vi "serialPorts.vi"(8 "list?":bool=TRUE, 11 "Python version":string) -> (0 "error out":errorcluster, 1 "ports":string[](array[string]), 2 "appended path":path, 3 "Refnum out":refnum<k35>)   [LabVIEW 2021]
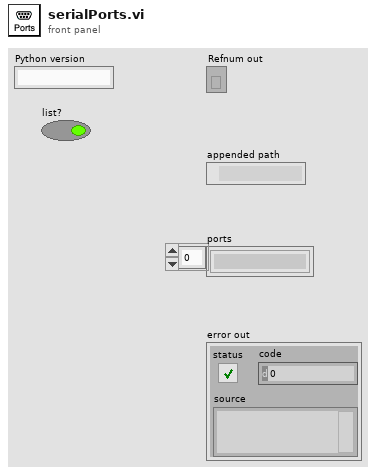
[diagram p1: front panel]
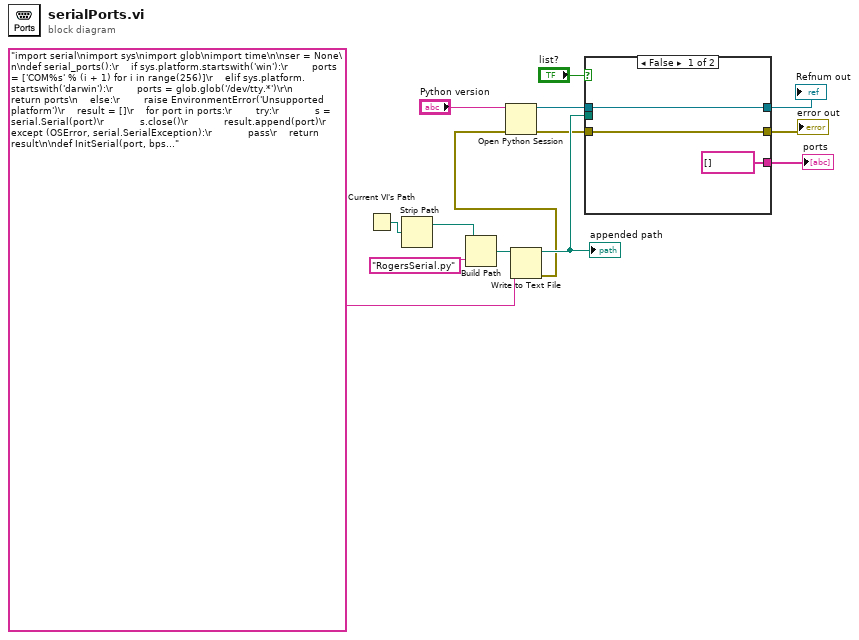
[diagram p0: block diagram]
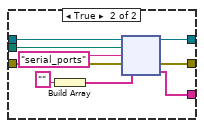
[diagram p2: hidden frame]
diagram:
  n1 = Current VI's Path() -> (path=w7:path)
  n2 = Strip Path(path=w7) -> (stripped path=w8:path)  [unwired: 1 out]
  n3 = Build Path(base path=w8, name or relative path="RogersSerial.py") -> (appended path=w13:path)
  "appended path" <- w13
  n4 = Write to Text File(file (use dialog)=w13, text="import serial\nimport sys\nimport glob\nimport time\n\nser = None\n\ndef serial_ports():\r    if sys.platform.startswith('win'):\r        ports = ['COM%s' % (i + 1) for i in range(256)]\r    elif sys.platform.startswith('darwin'):\r        ports = glob.glob('/dev/tty.*')\r\n        return ports\n    else:\r        raise EnvironmentError('Unsupported platform')\r    result = []\r    for port in ports:\r        try:\r            s = serial.Serial(port)\r            s.close()\r            result.append(port)\r        except (OSError, serial.SerialException):\r            pass\r    return result\n\ndef InitSerial(port, bps = 9600, to = 0):\n    global ser\n    ser = serial.Serial(port, bps, timeout = to)  # open serial port\n    ser.flushInput()\n    ser.flushOutput()\n    return ser.name\n\ndef FlushSerial():\n    ser.flushInput()\n    ser.flushOutput()\n    return(ser.in_waiting)\n\ndef CloseSerial():\n    ser.flush()\n    ser.close()\n    return('done')\n\ndef WriteSerial(string):\n    return (ser.write(string.encode()))    # write a string\n\ndef WriteBytes(data,replyLength):\n    buffer=ser.read(ser.in_waiting)\n    reply = ser.write(bytes(data))\n    if (replyLength < 0): return []\n    return list(ser.read(replyLength))    # write bytes and get reply\n\ndef ScriptSerial(string):\n    reply = ''\n    lines = string.split('\\n')\n    for line in lines:\n        ser.write(line.encode())\n        time.sleep(1)\n        reply += ReadSerial() + '\\n'\n    return reply \n\ndef ReadSerial():\n    reply = ''\n    if ser.in_waiting:\n        reply = ser.readline().decode()\n    return(reply)\n\n# note if the timeout is anything but zero it is slow") -> (error out=w3:errorcluster)  [unwired: 2 in, 2 out]
  n5 = Open Python Session(python version="Python version", 3:w3) -> (session out=w12:refnum<k35>, error out=w2:errorcluster)  [unwired: 1 in]
  n6 = case shown="False" "list?" {
    tunnel: w13 -> [_ w25]
    tunnel: w12 -> [w16 w24]
    tunnel: [w15 w23] -> w11
    tunnel: [string[] [] w22] -> w10
    tunnel: [w16 w18] -> w4
    tunnel: w2 -> [w15 w17]
    frame False {
    }
    frame True {
      n7 = Build Array("" ("function name")) -> (w21:string[])
      n8 = node(w24, w25, "serial_ports" ("function name"), w17, w21) -> (w18:refnum<k35>, w23:errorcluster, w22:string[])  [unwired: 2 out]
    }
  }
  "Refnum out" <- w4
  "error out" <- w11
  "ports" <- w10
